vi "Delta init.vi"(4 "Delta Mode Params In":T1={"High Level (A)"=0.001, "Low Level (A)"=-0.001, "Delay (s)"=0.002, "Num Cycles Mode"=enum."Infinite", "Finite Count"=10, "Abort On\nCompliance?"=FALSE, "Cold Swithing\nMode Enabled?"=FALSE} {"Finite Count" min=2 max=65536; "Low Level (A)" min=-0.105 max=0.0 format="%.3p"; "High Level (A)" min=0.0 max=0.105 format="%.3p"; "Delay (s)" min=0.001 max=9999.999 format="%.3f"}, 5 "2812 -A Params In":T12={"Auto Range?"=FALSE, "Man / Selected\nRange"=enum."10mV", "Enable Digital\nFilter?"=FALSE, "Filter Type"=enum."Moving", "Filter Count"=10, "Filter\nWindow (%)"=0.01, "Enable Analog\nFilter?"=FALSE, "NPLCs"=2} {"Filter\nWindow (%)" min=0.0 max=10.0 step=0.01 format="%.2f"; "Filter Count" min=1 max=100; "NPLCs" min=1 max=10}, 6 "Voltage Meas Units":T13, 7 "VISA Refnum in":refnum<visa-resource-name>="GPIB0::12::INSTR") -> (0 "error out":errorcluster, 3 "VISA Refnum out":refnum<visa-resource-name>)   [LabVIEW 2023]
uses:
  <instrlib>/Keithley 622x LV 2009/Configure/Units/Typedefs/KE622x -- Voltage Meas Units.ctl
  <instrlib>/Keithley 622x LV 2009/Configure/2182 -A/Low Level/Typedefs/KE2182 -- Voltage Ranges.ctl
  <instrlib>/Keithley 622x LV 2009/Configure/2182 -A/Low Level/Typedefs/KE2182 -- Filter Type.ctl
  <instrlib>/Keithley 622x LV 2009/Configure/2182 -A/Low Level/Typedefs/KE2182 -- Filter Count.ctl
  <instrlib>/Keithley 622x LV 2009/Configure/2182 -A/Low Level/Typedefs/KE2182 -- Filter Window.ctl
  <instrlib>/Keithley 622x LV 2009/Configure/2182 -A/Low Level/Typedefs/KE2182 -- NPLCs.ctl
  <instrlib>/Keithley 622x LV 2009/Configure/Delta PDelta DCon Modes/Typedefs/KE622x -- Delta Mode Params.ctl
  <instrlib>/Keithley 622x LV 2009/Configure/Delta PDelta DCon Modes/Low Level/Typedefs/KE622x -- Delta PDelta Mode High Level.ctl
  <instrlib>/Keithley 622x LV 2009/Configure/Delta PDelta DCon Modes/Low Level/Typedefs/KE622x -- Delta PDelta Mode Low Level.ctl
  <instrlib>/Keithley 622x LV 2009/Configure/Delta PDelta DCon Modes/Low Level/Typedefs/KE622x -- Delta DCon Mode Delay.ctl
  <instrlib>/Keithley 622x LV 2009/Configure/Delta PDelta DCon Modes/Low Level/Typedefs/KE622x -- Delta PDelta Mode Num Cycles Mode.ctl
  <instrlib>/Keithley 622x LV 2009/Configure/Delta PDelta DCon Modes/Low Level/Typedefs/KE622x -- Delta PDelta Mode Num Cycles.ctl
  <instrlib>/Keithley 622x LV 2009/Action-Status/Typedefs/KE622x -- Math Result Type.ctl
  <instrlib>/Keithley 622x LV 2009/Keithley 622x.lvlib
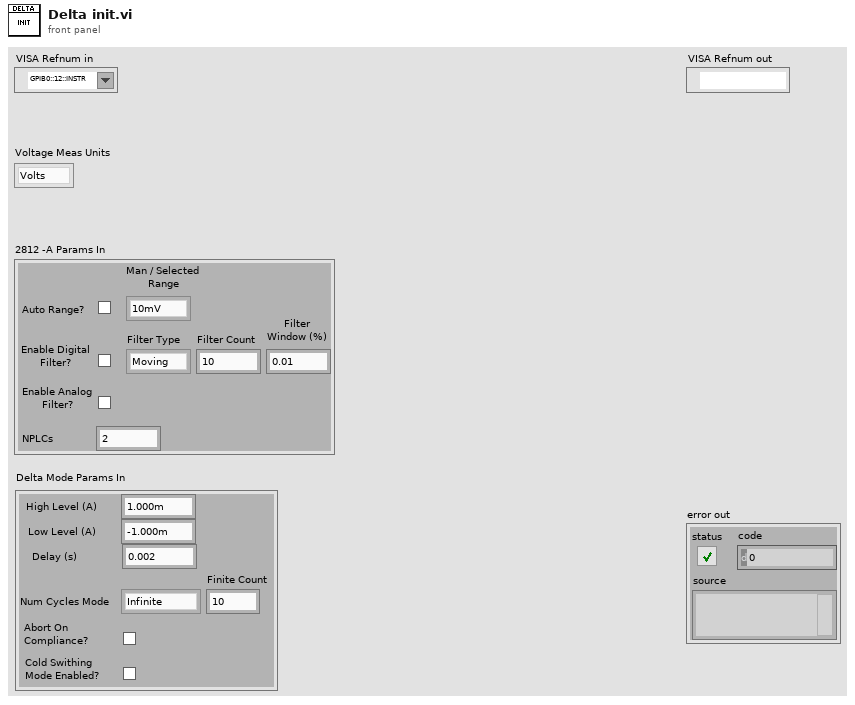
[diagram p1: front panel]
types:
  T1 = typedef "Keithley 622x.lvlib/KE622x -- Delta Mode Params.ctl" = cluster{"High Level (A)":T2, "Low Level (A)":T3, "Delay (s)":T4, "Num Cycles Mode":T5, "Finite Count":T6, "Abort On\nCompliance?":bool, "Cold Swithing\nMode Enabled?":bool}
  T2 = typedef "Keithley 622x.lvlib/KE622x -- Delta PDelta Mode High Level.ctl" = dbl
  T3 = typedef "Keithley 622x.lvlib/KE622x -- Delta PDelta Mode Low Level.ctl" = dbl
  T4 = typedef "Keithley 622x.lvlib/KE622x -- Delta DCon Mode Delay.ctl" = dbl
  T5 = typedef "Keithley 622x.lvlib/KE622x -- Delta PDelta Mode Num Cycles Mode.ctl" = enum16{"Finite Count", "Infinite"}
  T6 = typedef "Keithley 622x.lvlib/KE622x -- Delta PDelta Mode Num Cycles.ctl" = u32
  T7 = typedef "Keithley 622x.lvlib/KE2182 -- Voltage Ranges.ctl" = enum16{"10mV", "100mV", "1V", "10V", "100V"}
  T8 = typedef "Keithley 622x.lvlib/KE2182 -- Filter Type.ctl" = enum16{"Moving", "Repeat"}
  T9 = typedef "Keithley 622x.lvlib/KE2182 -- Filter Count.ctl" = u32
  T10 = typedef "Keithley 622x.lvlib/KE2182 -- Filter Window.ctl" = dbl
  T11 = typedef "Keithley 622x.lvlib/KE2182 -- NPLCs.ctl" = u32
  T12 = cluster{"Auto Range?":bool, "Man / Selected\nRange":T7, "Enable Digital\nFilter?":bool, "Filter Type":T8, "Filter Count":T9, "Filter\nWindow (%)":T10, "Enable Analog\nFilter?":bool, "NPLCs":T11}
  T13 = typedef "Keithley 622x.lvlib/KE622x -- Voltage Meas Units.ctl" = enum16{"Volts", "Ohms", "Watts", "Siemens"}
  T14 = typedef "Keithley 622x.lvlib/KE622x -- Math Result Type.ctl" = enum16{"Latest", "Fresh"}
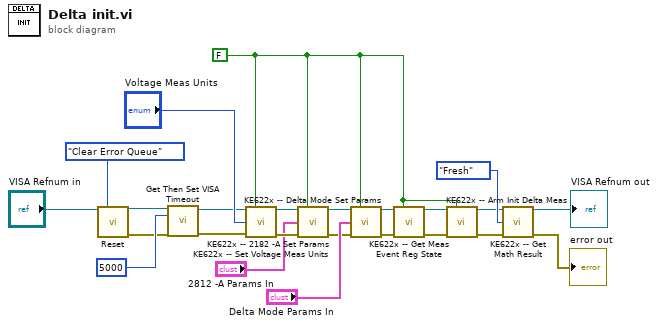
[diagram p0: block diagram]
diagram:
  w15 = FALSE
  n1 = call <instrlib>:"Reset.vi"("VISA resource name"="VISA Refnum in", "Error Queue Option"=enum16{"Clear Error Queue", "Error Query"}."Clear Error Queue") -> ("VISA resource name out"=w1:refnum<visa-resource-name>, "error out"=w4:errorcluster)  [unwired: 12 in]
  n2 = call <instrlib>:"Get Then Set VISA Timeout.vi"("VISA Resource Name In"=w1, "New Timeout (msecs)"=u32 5000, "error in (no error)"=w4) -> ("VISA Resource Name Out (dupl)"=w2:refnum<visa-resource-name>, "error out"=w3:errorcluster)  [unwired: 9 in, 2 out]
  n3 = call <instrlib>:"KE622x -- Set Voltage Meas Units.vi"("Resource In"=w2, "Check For SCPI Errors? (T)"=w15, "Voltage Meas Units"="Voltage Meas Units", "error in (no error)"=w3) -> ("Resource Out (dupl)"=w21:refnum<visa-resource-name>, "error out"=w22:errorcluster)  [unwired: 10 in]
  n4 = call <instrlib>:"KE622x -- 2182 -A Set Params.vi"("622x Resource In"=w21, "Check For SCPI Errors? (T)"=w15, "2812 -A Params In"="2812 -A Params In", "error in (no error)"=w22) -> ("622x Resource Out (dupl)"=w10:refnum<visa-resource-name>, "error out"=w11:errorcluster)  [unwired: 9 in, 1 out]
  n5 = call <instrlib>:"KE622x -- Delta Mode Set Params.vi"("Resource In"=w10, "Check For SCPI Errors? (T)"=w15, "Delta Mode Params In"="Delta Mode Params In", "error in (no error)"=w11) -> ("Resource Out (dupl)"=w23:refnum<visa-resource-name>, "error out"=w24:errorcluster)  [unwired: 9 in, 1 out]
  n6 = call <instrlib>:"KE622x -- Get Meas Event Reg State.vi"("VISA Resource In"=w23, "Error Query (T)?"=w15, "error in (no error)"=w24) -> ("VISA Resource Out (dupl)"=w13:refnum<visa-resource-name>, "error out"=w14:errorcluster)  [unwired: 10 in, 1 out]
  n7 = call <instrlib>:"KE622x -- Arm Init Delta Meas.vi"("Resource In"=w13, "Check For SCPI Errors? (T)"=w15, "error in (no error)"=w14) -> ("Resource Out (dupl)"=w19:refnum<visa-resource-name>, "error out"=w18:errorcluster)  [unwired: 11 in]
  n8 = call <instrlib>:"KE622x -- Get Math Result.vi"("Resource In"=w19, "Result Type"=KE622x_--_Math_Result_Type."Fresh", "error in (no error)"=w18) -> ("Resource Out (dupl)"=→"VISA Refnum out":refnum<visa-resource-name>, "error out"=→"error out":errorcluster)  [unwired: 10 in, 1 out]
